vi "Get Added Plot Index.vi"(8 "Plot Index (Append)":i32=2147483647, 10 "Graph # Plots":i32) -> (0 "Actual Plot Index":i32, 3 "Append to End?":bool)   [LabVIEW 2021, in "Graphs.lvlib"]
doc: "Check whether the plot to add to a graph overwrites an existing one or is appended to the end (default).\n\nDefault Plot Index: 2,147,483,648 (= Inf) == Append to End\nNegative Plot Indices are counted from the last plot (-1: last, -2: next to last, etc.)"
uses:
  Graphs.lvlib
  Math/Math.lvlib
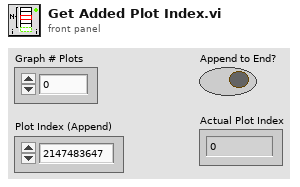
[diagram p1: front panel]
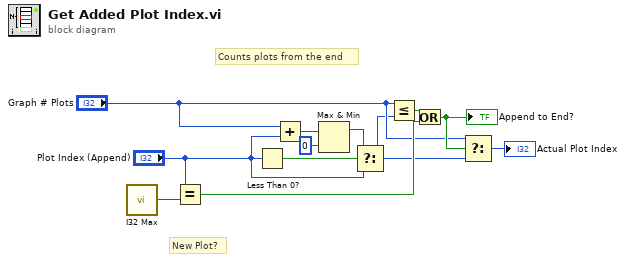
[diagram p0: block diagram]
diagram:
  # "Counts plots from the end"
  # "New Plot?"
  n1 = call "I32 Max.vi"() -> ("I32 max"=w7:i32)
  n2 = Equal?(x="Plot Index (Append)", y=w7) -> (x = y?=w5:bool)
  n3 = Less Than 0?(x="Plot Index (Append)") -> (x < 0?=w9:bool)
  n4 = Add(x="Graph # Plots", y="Plot Index (Append)") -> (x+y=w12:i32)
  n5 = Max & Min(x=w12, y=0) -> (max(x,y)=w11:i32)  [unwired: 1 out]
  n6 = Select(t=w11, s=w9, f="Plot Index (Append)") -> (s? t:f=w2:i32)
  n7 = Less Or Equal?(x="Graph # Plots", y=w2) -> (x <= y?=w6:bool)
  n8 = Or(x=w6, y=w5) -> (x .or. y?=w4:bool)
  "Append to End?" <- w4
  n9 = Select(t="Graph # Plots", s=w4, f=w2) -> (s? t:f=→"Actual Plot Index":i32)
